vi "H5Pset_szip.vi"(6 "error in (no error)":errorcluster, 7 "Pixels per block":u32=8 min=2 max=32 step=2, 8 "SZip Options":T1 items=["H5_SZIP_NO_OPTIONS"=0, "H5_SZIP_ALLOW_K13_OPTION_MASK"=1, "H5_SZIP_CHIP_OPTION_MASK"=2, "H5_SZIP_EC_OPTION_MASK"=4, "H5_SZIP_NN_OPTION_MASK"=32], 9 "HDF5 Property Ref":T2) -> (0 "error out":errorcluster, 3 "HDF5 Ref out":T2)   [LabVIEW 2017]
doc: "Sets up use of the SZIP compression filter."
uses:
  <vilib>/UPVI/lvhdf5/library.llb/HDF5 Ref.ctl
  <vilib>/UPVI/lvhdf5/property.llb/H5_szip_options_t.ctl
  <vilib>/UPVI/lvhdf5/hdf5.dll
panel:
  # "LVHDF5 Toolkit\nCopyright (c) 2005-2013 by Jason D. Sommerville\nCopyright (c) 2014 by UPVI, LLC.\n\nThis use and distribution of this file is governed by the terms found in \nLICENSE.txt distributed with this toolkit and installed at\n <user.lib>\\_lvhdf5\\LICENSE.txt"
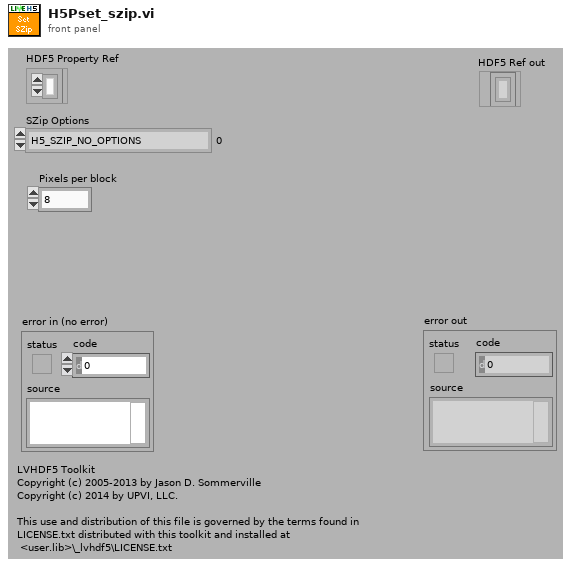
[diagram p1: front panel]
types:
  T1 = typedef "H5_szip_options_t.ctl" = u32
  T2 = typedef "HDF5 Ref.ctl" = refnum<k1>
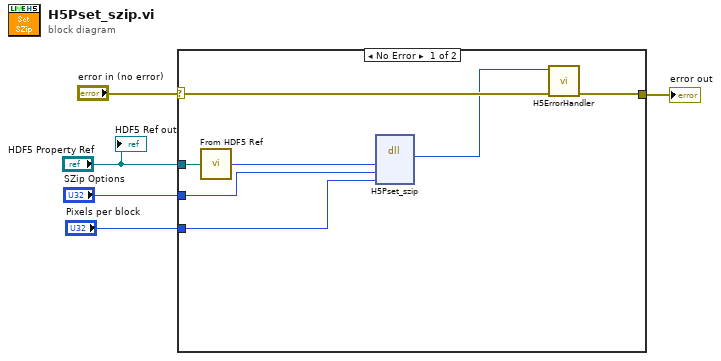
[diagram p0: block diagram]
diagram:
  n1 = case shown="No Error" "error in (no error)" {
    selector: "error in (no error)" -> [w12 w13]
    tunnel: [w11 w13] -> w4
    tunnel: "HDF5 Property Ref" -> [w9 _]
    tunnel: "SZip Options" -> [w7 _]
    tunnel: "Pixels per block" -> [w6 _]
    frame No Error {
      n2 = call <vilib>:"From HDF5 Ref.vi"("HDF5 Ref"=w9) -> ("I32"=w8:i32)
      n3 = dll-call lib="C:/Program Files/National Instruments/LabVIEW 2017/vi.lib/UPVI/lvhdf5/hdf5.dll" fn="H5Pset_szip"("plist_id"=w8, "options"=w7, "pixels_per_block"=w6) -> (w10:i32)  [unwired: 6 in, 2 out]
      n4 = call <vilib>:"H5ErrorHandler.vi"("error in (no error)"=w12, "herr_t"=w10) -> ("error out"=w11:errorcluster)  [unwired: 3 in, 4 out]
    }
    frame Error {
    }
  }
  "error out" <- w4
  "HDF5 Ref out" <- "HDF5 Property Ref"
